vi "File_header_diag.vi"(8 "Preparation time":timestamp, 9 "Time resolved?":bool, 10 "Comment":string, 11 "Byte Stream File in":refnum<file>) -> ()   [LabVIEW 2013]
uses:
  <vilib>/Utility/file.llb/Write To Spreadsheet File (string).vi
panel:
  out "resulting string":string
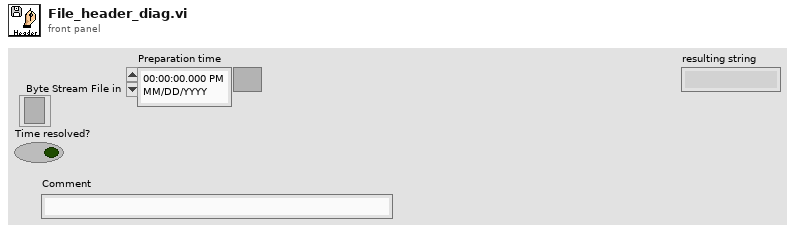
[diagram p1: front panel]
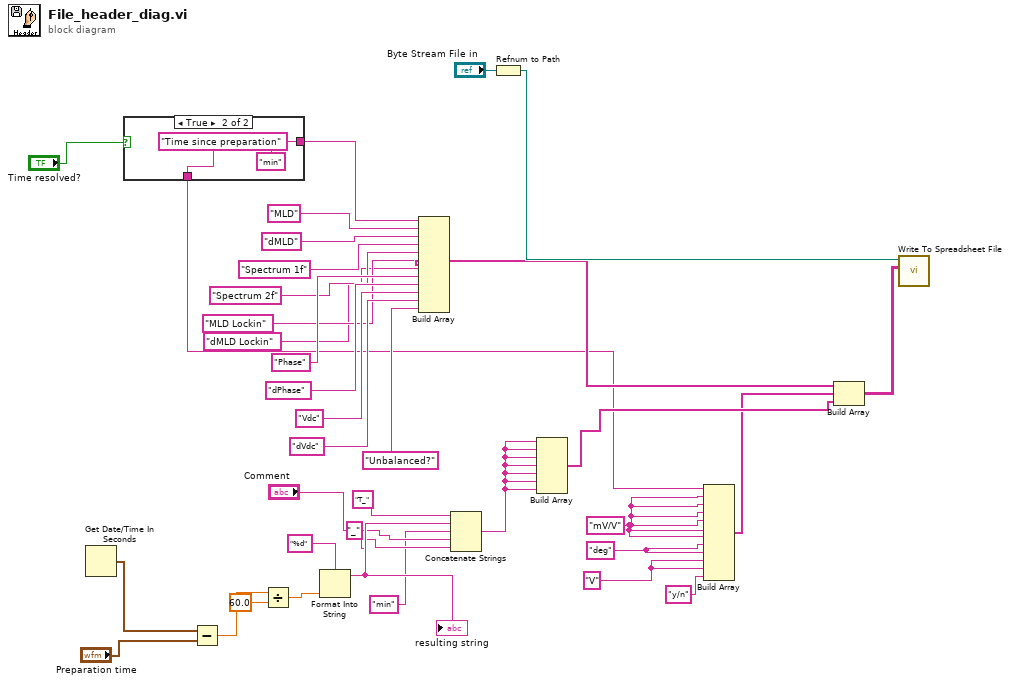
[diagram p0: block diagram]
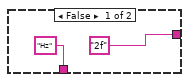
[diagram p2: hidden frame]
diagram:
  w4 = "V"
  w6 = "deg"
  w5 = "mV/V"
  n1 = Get Date/Time In Seconds() -> (seconds since 1Jan1904=w12:timestamp)
  n2 = case shown="True" "Time resolved?" {
    tunnel: ["2f" "Time since preparation"] -> w33
    tunnel: ["Hz" "min"] -> w1
    frame False {
    }
    frame True {
    }
  }
  n3 = Subtract(x=w12, y="Preparation time") -> (x-y=w19:dbl)
  n4 = Divide(x=w19, y=60.0) -> (x/y=w17:dbl)
  n5 = Format Into String(format string="%d", w17) -> (resulting string=w13:string)  [unwired: 2 in, 1 out]
  "resulting string" <- w13
  n6 = Build Array(w33, "MLD", "dMLD", "Spectrum 1f", "Spectrum 2f", "MLD Lockin", "dMLD Lockin", "Phase", "dPhase", "Vdc", "dVdc", "Unbalanced?" ("element")) -> (w26:string[])
  n7 = Concatenate Strings("T_" ("string"), w13, "min" ("string"), "_" ("string"), "Comment") -> (w15:string)
  n8 = Refnum to Path(1:"Byte Stream File in") -> (0:w35:path)
  n9 = Build Array(w15, w15, w15, w15, w15, w15, w15) -> (w7:string[])
  n10 = Build Array(w1, w5, w5, w5, w5, w5, w5, w6, w6, w4, w4, "y/n" ("element")) -> (w2:string[])
  n11 = Build Array(w26, w2, w7) -> (w34:string[][])
  n12 = call-poly <vilib>:"Write To Spreadsheet File.vi"("2D data"=w34, "file path (dialog if empty)"=w35) -> ()  [unwired: 6 in, 1 out]
